vi "set_minimum_and_maximum.vi"(8 "error in (no error)":errorcluster, 9 "maximum":refnum<class "SpaceVector.lvclass">, 10 "minimum":refnum<class "SpaceVector.lvclass">, 11 "Box in":refnum<class "Box.lvclass">) -> (0 "error out":errorcluster, 3 "Box out":refnum<class "Box.lvclass">)   [LabVIEW 2010, in "Box.lvclass"]
uses:
  Box.lvclass
  SpaceVector/SpaceVector/SpaceVector.lvclass
  Box.lvclass/Box.ctl
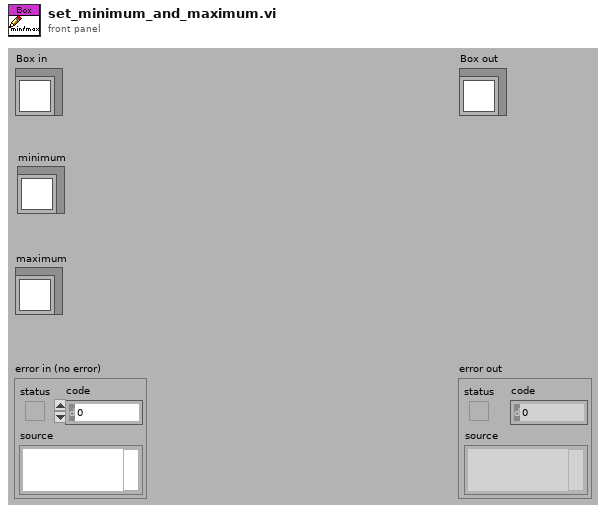
[diagram p1: front panel]
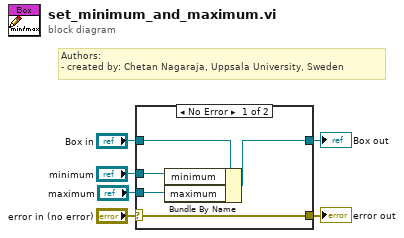
[diagram p0: block diagram]
diagram:
  # "Authors: \n- created by: Chetan Nagaraja, Uppsala University, Sweden"
  n1 = case shown="No Error" "error in (no error)" {
    selector: "error in (no error)" -> [w11 w13]
    tunnel: [w11 w13] -> w5
    tunnel: [w9 w12] -> w3
    tunnel: "Box in" -> [w10 w12]
    tunnel: "minimum" -> [w8 _]
    tunnel: "maximum" -> [w7 _]
    frame No Error {
      n2 = Bundle By Name(cluster=w10, "minimum"=w8, "maximum"=w7) -> (w9:refnum<class "Box.lvclass">)
    }
    frame Error {
    }
  }
  "error out" <- w5
  "Box out" <- w3
